vi "Init_Instr.vi"(8 "error in (no error)":errorcluster caption="entrée d'erreur (pas d'erreur)", 11 "Class DIO en entrée":refnum<class "Class Instrument DIO.lvclass">) -> (0 "error out":errorcluster caption="sortie d'erreur", 3 "Class DIO en Sortie":refnum<class "Class Instrument DIO.lvclass">)   [LabVIEW 2020, in "Library Instrument & Equipement.lvlib" / "Library Instruments.lvlib" / "Class Instrument DIO.lvclass"]
uses:
  Class Instrument DIO.lvclass
  Class Instrument DIO.lvclass/Class Instrument DIO.ctl
  Instrument (Default)/Class Instrument (Default).lvclass
  DIO/Class DIO (Default)/Class DIO (Default).lvclass
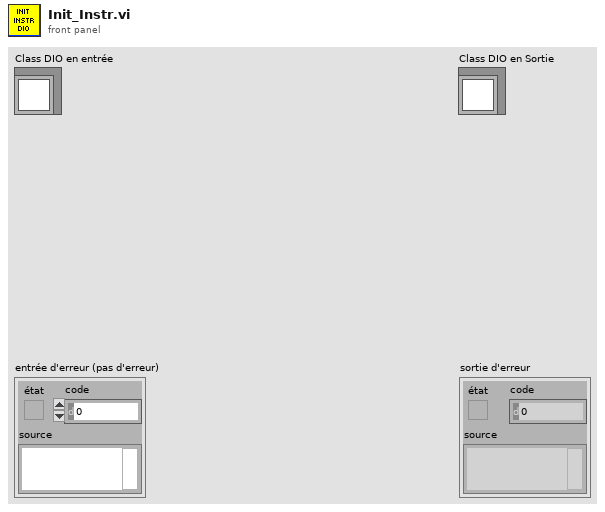
[diagram p1: front panel]
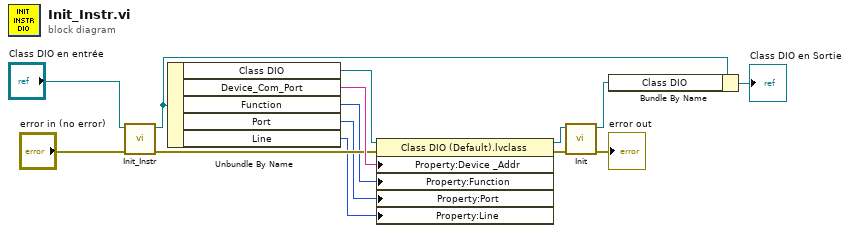
[diagram p0: block diagram]
diagram:
  n1 = call-parent "Init_Instr.vi"("error in (no error)"="error in (no error)", "Class Instrument (Default) en entrée"="Class DIO en entrée") -> ("error out"=w10:errorcluster, "Class Instrument (Default) en sortie"=w9:refnum<class "Class Instrument DIO.lvclass">)  [unwired: 8 in]
  n2 = Unbundle By Name(w9) -> ("Class DIO"=w12:refnum<class "Class DIO (Default).lvclass">, "Device_Com_Port"=w11:string, "Function"=w8:enum16{"Write", "Read"}, "Port"=w7:u8, "Line"=w6:u8)
  n3 = property class="Class DIO (Default).lvclass"(reference=w12, error in=w10, "Property:Device _Addr"=w11, "Property:Function"=w8, "Property:Port"=w7, "Property:Line"=w6) -> (reference out=w4:refnum<class "Class DIO (Default).lvclass">, error out=w5:errorcluster)
  n4 = call-dynamic "Init.vi"("error in (no error)"=w5, "Class DIO (Default) en entrée"=w4) -> ("error out"=→"error out":errorcluster, "Class DIO (Default) en sortie"=w3:refnum<class "Class DIO (Default).lvclass">)  [unwired: 8 in]
  n5 = Bundle By Name(cluster=w9, "Class DIO"=w3) -> (→"Class DIO en Sortie":refnum<class "Class Instrument DIO.lvclass">)
